vi "input_channel_task.vi"(8 "error in":errorcluster, 10 "Analog Input Channels":T2[](array[typedef])=[{"Input Type"=enum."DAQ", "Channel Name"="Vapor Mass Flow", "Physical Channel"="cDAQ1Mod2/ai5", "Sensor Type"=enum."Mass Flow Rate", "Signal Type"=enum."Current", "Terminal Configuration"=-1, "Minimum Value"=0.004, "Maximum Value"=0.02, "TC Type"=10086, "Sensor Min"=0.0, "Sensor Max"=377.9933, "Sensor Offset"=0.0, "Sensor Unit"=enum."g/s", "Output Unit"=enum."g/s", "Unit Conversion"=1.0, "Active"=TRUE}, {"Input Type"=enum."DAQ", "Channel Name"="Vapor Line Density", "Physical Channel"="cDAQ1Mod2/ai6", "Sensor Type"=enum."Density", "Signal Type"=enum."Current", "Terminal Configuration"=-1, "Minimum Value"=0.004, "Maximum Value"=0.02, "TC Type"=10086, "Sensor Min"=0.0, "Sensor Max"=2.0, "Sensor Offset"=0.0, "Sensor Unit"=enum."g/cm3", "Output Unit"=enum."g/cm3", "Unit Conversion"=1.0, "Active"=TRUE}, {"Input Type"=enum."DAQ", "Channel Name"="Liquid Mass Flow", "Physical Channel"="cDAQ1Mod2/ai3", "Sensor Type"=enum."Mass Flow Rate", "Signal Type"=enum."Current", "Terminal Configuration"=-1, "Minimum Value"=0.004, "Maximum Value"=0.02, "TC Type"=10086, "Sensor Min"=0.0, "Sensor Max"=377.9933, "Sensor Offset"=0.0, "Sensor Unit"=enum."g/s", "Output Unit"=enum."g/s", "Unit Conversion"=1.0, "Active"=TRUE}, {"Input Type"=enum."DAQ", "Channel Name"="Liquid Line Density", "Physical Channel"="cDAQ1Mod2/ai4", "Sensor Type"=enum."Density", "Signal Type"=enum."Current", "Terminal Configuration"=-1, "Minimum Value"=0.004, "Maximum Value"=0.02, "TC Type"=10086, "Sensor Min"=0.0, "Sensor Max"=2.0, "Sensor Offset"=0.0, "Sensor Unit"=enum."g/cm3", "Output Unit"=enum."g/cm3", "Unit Conversion"=1.0, "Active"=TRUE}, {"Input Type"=enum."DAQ", "Channel Name"="Vapor Inlet Pressure DEPR", "Physical Channel"="cDAQ1Mod5/ai1", "Sensor Type"=enum."Absolute Pressure", "Signal Type"=enum."Voltage", "Terminal Configuration"=10078, "Minimum Value"=0.0, "Maximum Value"=5.0, "TC Type"=10086, "Sensor Min"=0.0, "Sensor Max"=50.0, "Sensor Offset"=0.0, "Sensor Unit"=enum."psi", "Output Unit"=enum."Pa", "Unit Conversion"=6894.75729, "Active"=FALSE}, {"Input Type"=enum."DAQ", "Channel Name"="Mega Tank Pressure", "Physical Channel"="cDAQ1Mod5/ai2", "Sensor Type"=enum."Absolute Pressure", "Signal Type"=enum."Voltage", "Terminal Configuration"=10078, "Minimum Value"=0.5, "Maximum Value"=5.5, "TC Type"=10086, "Sensor Min"=0.0, "Sensor Max"=50.0, "Sensor Offset"=0.0, "Sensor Unit"=enum."psi", "Output Unit"=enum."Pa", "Unit Conversion"=6894.75729, "Active"=TRUE}, {"Input Type"=enum."DAQ", "Channel Name"="Separator Pressure", "Physical Channel"="cDAQ1Mod5/ai0", "Sensor Type"=enum."Absolute Pressure", "Signal Type"=enum."Voltage", "Terminal Configuration"=10078, "Minimum Value"=0.0, "Maximum Value"=5.0, "TC Type"=10086, "Sensor Min"=0.0, "Sensor Max"=50.0, "Sensor Offset"=0.0, "Sensor Unit"=enum."psi", "Output Unit"=enum."Pa", "Unit Conversion"=6894.75729, "Active"=TRUE}, {"Input Type"=enum."DAQ", "Channel Name"="Liquid Inlet Pressure", "Physical Channel"="cDAQ1Mod5/ai4", "Sensor Type"=enum."Absolute Pressure", "Signal Type"=enum."Voltage", "Terminal Configuration"=10078, "Minimum Value"=0.0, "Maximum Value"=5.0, "TC Type"=10086, "Sensor Min"=0.0, "Sensor Max"=50.0, "Sensor Offset"=0.0, "Sensor Unit"=enum."psi", "Output Unit"=enum."Pa", "Unit Conversion"=6894.75729, "Active"=TRUE}, {"Input Type"=enum."DAQ", "Channel Name"="Vapor Inlet Pressure ", "Physical Channel"="cDAQ1Mod5/ai3", "Sensor Type"=enum."Absolute Pressure", "Signal Type"=enum."Voltage", "Terminal Configuration"=10078, "Minimum Value"=0.0, "Maximum Value"=5.0, "TC Type"=10086, "Sensor Min"=0.0, "Sensor Max"=50.0, "Sensor Offset"=0.0, "Sensor Unit"=enum."psi", "Output Unit"=enum."Pa", "Unit Conversion"=6894.75729, "Active"=TRUE}, {"Input Type"=enum."DAQ", "Channel Name"="Vapor Inlet Temperature", "Physical Channel"="cDAQ1Mod6/ai1", "Sensor Type"=enum."Temperature", "Signal Type"=enum."Temperature", "Terminal Configuration"=-1, "Minimum Value"=0.0, "Maximum Value"=100.0, "TC Type"=10086, "Sensor Min"=0.0, "Sensor Max"=100.0, "Sensor Offset"=0.0, "Sensor Unit"=enum."C", "Output Unit"=enum."C", "Unit Conversion"=1.0, "Active"=TRUE}, {"Input Type"=enum."DAQ", "Channel Name"="Vapor Inlet Temperature DEPR", "Physical Channel"="cDAQ1Mod7/ai0", "Sensor Type"=enum."Temperature", "Signal Type"=enum."Temperature", "Terminal Configuration"=-1, "Minimum Value"=0.0, "Maximum Value"=100.0, "TC Type"=10086, "Sensor Min"=0.0, "Sensor Max"=100.0, "Sensor Offset"=0.0, "Sensor Unit"=enum."C", "Output Unit"=enum."C", "Unit Conversion"=1.0, "Active"=FALSE}, {"Input Type"=enum."DAQ", "Channel Name"="Mega Tank Temperature", "Physical Channel"="cDAQ1Mod6/ai2", "Sensor Type"=enum."Temperature", "Signal Type"=enum."Temperature", "Terminal Configuration"=-1, "Minimum Value"=0.0, "Maximum Value"=100.0, "TC Type"=10086, "Sensor Min"=0.0, "Sensor Max"=100.0, "Sensor Offset"=0.0, "Sensor Unit"=enum."C", "Output Unit"=enum."C", "Unit Conversion"=1.0, "Active"=TRUE}, {"Input Type"=enum."DAQ", "Channel Name"="Liquid Inlet Temperature", "Physical Channel"="cDAQ1Mod7/ai3", "Sensor Type"=enum."Temperature", "Signal Type"=enum."Temperature", "Terminal Configuration"=-1, "Minimum Value"=0.0, "Maximum Value"=100.0, "TC Type"=10086, "Sensor Min"=0.0, "Sensor Max"=100.0, "Sensor Offset"=0.0, "Sensor Unit"=enum."C", "Output Unit"=enum."C", "Unit Conversion"=1.0, "Active"=TRUE}, {"Input Type"=enum."DAQ", "Channel Name"="Separator Temperature", "Physical Channel"="cDAQ1Mod6/ai0", "Sensor Type"=enum."Temperature", "Signal Type"=enum."Temperature", "Terminal Configuration"=-1, "Minimum Value"=0.0, "Maximum Value"=100.0, "TC Type"=10086, "Sensor Min"=0.0, "Sensor Max"=100.0, "Sensor Offset"=0.0, "Sensor Unit"=enum."C", "Output Unit"=enum."C", "Unit Conversion"=1.0, "Active"=TRUE}, {"Input Type"=enum."DAQ", "Channel Name"="Lower Dev Section Pressure", "Physical Channel"="cDAQ1Mod5/ai6", "Sensor Type"=enum."Absolute Pressure", "Signal Type"=enum."Voltage", "Terminal Configuration"=10078, "Minimum Value"=0.0, "Maximum Value"=5.0, "TC Type"=10086, "Sensor Min"=0.0, "Sensor Max"=60.0, "Sensor Offset"=0.0, "Sensor Unit"=enum."psi", "Output Unit"=enum."Pa", "Unit Conversion"=6894.75729, "Active"=TRUE}, {"Input Type"=enum."DAQ", "Channel Name"="Upper Dev Section Temperature", "Physical Channel"="cDAQ1Mod6/ai3", "Sensor Type"=enum."Temperature", "Signal Type"=enum."Temperature", "Terminal Configuration"=-1, "Minimum Value"=0.0, "Maximum Value"=100.0, "TC Type"=10086, "Sensor Min"=0.0, "Sensor Max"=100.0, "Sensor Offset"=0.0, "Sensor Unit"=enum."C", "Output Unit"=enum."C", "Unit Conversion"=1.0, "Active"=TRUE}, {"Input Type"=enum."DAQ", "Channel Name"="Upper Dev Section Pressure", "Physical Channel"="cDAQ1Mod5/ai5", "Sensor Type"=enum."Absolute Pressure", "Signal Type"=enum."Voltage", "Terminal Configuration"=10078, "Minimum Value"=0.0, "Maximum Value"=5.0, "TC Type"=10086, "Sensor Min"=0.0, "Sensor Max"=60.0, "Sensor Offset"=0.0, "Sensor Unit"=enum."psi", "Output Unit"=enum."Pa", "Unit Conversion"=6894.75729, "Active"=TRUE}, {"Input Type"=enum."DAQ", "Channel Name"="Test Section Temperature", "Physical Channel"="cDAQ1Mod6/ai10", "Sensor Type"=enum."Temperature", "Signal Type"=enum."Temperature", "Terminal Configuration"=-1, "Minimum Value"=0.0, "Maximum Value"=100.0, "TC Type"=10086, "Sensor Min"=0.0, "Sensor Max"=100.0, "Sensor Offset"=0.0, "Sensor Unit"=enum."C", "Output Unit"=enum."C", "Unit Conversion"=1.0, "Active"=TRUE}, {"Input Type"=enum."DAQ", "Channel Name"="Test Section Pressure", "Physical Channel"="cDAQ1Mod5/ai7", "Sensor Type"=enum."Absolute Pressure", "Signal Type"=enum."Voltage", "Terminal Configuration"=10078, "Minimum Value"=0.0, "Maximum Value"=5.0, "TC Type"=10086, "Sensor Min"=0.0, "Sensor Max"=50.0, "Sensor Offset"=0.0, "Sensor Unit"=enum."psi", "Output Unit"=enum."Pa", "Unit Conversion"=6894.75729, "Active"=TRUE}, {"Input Type"=enum."DAQ", "Channel Name"="Dwyer dP DEPR", "Physical Channel"="cDAQ1Mod5/ai9", "Sensor Type"=enum."Differential Pressure", "Signal Type"=enum."Voltage", "Terminal Configuration"=10078, "Minimum Value"=0.05, "Maximum Value"=5.05, "TC Type"=10086, "Sensor Min"=0.0, "Sensor Max"=1.0, "Sensor Offset"=0.0, "Sensor Unit"=enum."psi", "Output Unit"=enum."Pa", "Unit Conversion"=6894.75729, "Active"=FALSE}, {"Input Type"=enum."DAQ", "Channel Name"="Venturi dP", "Physical Channel"="cDAQ1Mod9/ai0", "Sensor Type"=enum."Differential Pressure", "Signal Type"=enum."Current", "Terminal Configuration"=10083, "Minimum Value"=0.00403, "Maximum Value"=0.02, "TC Type"=10086, "Sensor Min"=0.0, "Sensor Max"=10.0, "Sensor Offset"=0.0, "Sensor Unit"=enum."inH2O", "Output Unit"=enum."Pa", "Unit Conversion"=248.84, "Active"=TRUE}, {"Input Type"=enum."DAQ", "Channel Name"="PGminiPressure", "Physical Channel"="cDAQ1Mod5/ai10", "Sensor Type"=enum."Absolute Pressure", "Signal Type"=enum."Voltage", "Terminal Configuration"=10078, "Minimum Value"=0.0, "Maximum Value"=5.0, "TC Type"=10086, "Sensor Min"=0.0, "Sensor Max"=50.0, "Sensor Offset"=0.0, "Sensor Unit"=enum."psi", "Output Unit"=enum."Pa", "Unit Conversion"=6894.75729, "Active"=TRUE}, {"Input Type"=enum."DAQ", "Channel Name"="PGminiTemperature", "Physical Channel"="cDAQ1Mod7/ai6", "Sensor Type"=enum."Temperature", "Signal Type"=enum."Temperature", "Terminal Configuration"=-1, "Minimum Value"=0.0, "Maximum Value"=100.0, "TC Type"=10073, "Sensor Min"=0.0, "Sensor Max"=100.0, "Sensor Offset"=0.0, "Sensor Unit"=enum."C", "Output Unit"=enum."C", "Unit Conversion"=1.0, "Active"=TRUE}, {"Input Type"=enum."DAQ", "Channel Name"="Atmospheric Pressure", "Physical Channel"="cDAQ1Mod5/ai8", "Sensor Type"=enum."Absolute Pressure", "Signal Type"=enum."Voltage", "Terminal Configuration"=10078, "Minimum Value"=1.0, "Maximum Value"=5.0, "TC Type"=10086, "Sensor Min"=0.0, "Sensor Max"=25.0, "Sensor Offset"=0.0, "Sensor Unit"=enum."psi", "Output Unit"=enum."Pa", "Unit Conversion"=6894.75729, "Active"=TRUE}, {"Input Type"=enum."DAQ", "Channel Name"="PG Absolute Pressure", "Physical Channel"="cDAQ1Mod5/ai11", "Sensor Type"=enum."Absolute Pressure", "Signal Type"=enum."Voltage", "Terminal Configuration"=10078, "Minimum Value"=0.0, "Maximum Value"=5.0, "TC Type"=10086, "Sensor Min"=0.0, "Sensor Max"=60.0, "Sensor Offset"=0.0, "Sensor Unit"=enum."psi", "Output Unit"=enum."Pa", "Unit Conversion"=6894.75729, "Active"=TRUE}, {"Input Type"=enum."DAQ", "Channel Name"="Dwyer dP", "Physical Channel"="cDAQ1Mod2/ai7", "Sensor Type"=enum."Differential Pressure", "Signal Type"=enum."Current", "Terminal Configuration"=-1, "Minimum Value"=0.004, "Maximum Value"=0.02, "TC Type"=10086, "Sensor Min"=0.0, "Sensor Max"=500.0, "Sensor Offset"=0.0, "Sensor Unit"=enum."Pa", "Output Unit"=enum."Pa", "Unit Conversion"=1.0, "Active"=TRUE}, {"Input Type"=enum."DAQ", "Channel Name"="Mixing Tee dP DEPR", "Physical Channel"="", "Sensor Type"=enum."Differential Pressure", "Signal Type"=enum."Current", "Terminal Configuration"=-1, "Minimum Value"=0.004, "Maximum Value"=0.02, "TC Type"=10086, "Sensor Min"=0.0, "Sensor Max"=50.0, "Sensor Offset"=0.0, "Sensor Unit"=enum."psi", "Output Unit"=enum."Pa", "Unit Conversion"=6894.75729, "Active"=FALSE}, {"Input Type"=enum."DAQ", "Channel Name"="PG Vapor Temperature", "Physical Channel"="cDAQ1Mod7/ai4", "Sensor Type"=enum."Temperature", "Signal Type"=enum."Temperature", "Terminal Configuration"=-1, "Minimum Value"=0.0, "Maximum Value"=100.0, "TC Type"=10073, "Sensor Min"=0.0, "Sensor Max"=100.0, "Sensor Offset"=0.0, "Sensor Unit"=enum."C", "Output Unit"=enum."C", "Unit Conversion"=1.0, "Active"=TRUE}, {"Input Type"=enum."DAQ", "Channel Name"="PG Liquid Temperature", "Physical Channel"="cDAQ1Mod7/ai5", "Sensor Type"=enum."Temperature", "Signal Type"=enum."Temperature", "Terminal Configuration"=-1, "Minimum Value"=0.0, "Maximum Value"=100.0, "TC Type"=10073, "Sensor Min"=0.0, "Sensor Max"=100.0, "Sensor Offset"=0.0, "Sensor Unit"=enum."C", "Output Unit"=enum."C", "Unit Conversion"=1.0, "Active"=TRUE}, {"Input Type"=enum."DAQ", "Channel Name"="Window 1 to 4 dP", "Physical Channel"="cDAQ1Mod2/ai2", "Sensor Type"=enum."Differential Pressure", "Signal Type"=enum."Current", "Terminal Configuration"=-1, "Minimum Value"=0.004, "Maximum Value"=0.02, "TC Type"=10086, "Sensor Min"=0.0, "Sensor Max"=20.0, "Sensor Offset"=0.0, "Sensor Unit"=enum."inH2O", "Output Unit"=enum."Pa", "Unit Conversion"=248.84, "Active"=TRUE}, {"Input Type"=enum."DAQ", "Channel Name"="Window 1 to 7 dP", "Physical Channel"="cDAQ1Mod2/ai1", "Sensor Type"=enum."Differential Pressure", "Signal Type"=enum."Current", "Terminal Configuration"=-1, "Minimum Value"=0.004, "Maximum Value"=0.02, "TC Type"=10086, "Sensor Min"=0.0, "Sensor Max"=20.0, "Sensor Offset"=0.0, "Sensor Unit"=enum."inH2O", "Output Unit"=enum."Pa", "Unit Conversion"=248.84, "Active"=TRUE}, {"Input Type"=enum."DAQ", "Channel Name"="Window 1 to 7 Fast dP", "Physical Channel"="cDAQ1Mod2/ai0", "Sensor Type"=enum."Differential Pressure", "Signal Type"=enum."Current", "Terminal Configuration"=-1, "Minimum Value"=0.004, "Maximum Value"=0.02, "TC Type"=10086, "Sensor Min"=0.0, "Sensor Max"=2.5, "Sensor Offset"=0.0, "Sensor Unit"=enum."psi", "Output Unit"=enum."Pa", "Unit Conversion"=6894.75729, "Active"=TRUE}, {"Input Type"=enum."DAQ", "Channel Name"="Camera Voltage", "Physical Channel"="cDAQ1Mod8/ai0", "Sensor Type"=enum."Other", "Signal Type"=enum."Voltage", "Terminal Configuration"=10106, "Minimum Value"=0.0, "Maximum Value"=10.0, "TC Type"=10086, "Sensor Min"=0.0, "Sensor Max"=50.0, "Sensor Offset"=0.0, "Sensor Unit"=enum."Volt", "Output Unit"=enum."Volt", "Unit Conversion"=1.0, "Active"=TRUE}, {"Input Type"=enum."DAQ", "Channel Name"="Tinlet", "Physical Channel"="cDAQ1Mod6/ai4", "Sensor Type"=enum."Temperature", "Signal Type"=enum."Temperature", "Terminal Configuration"=-1, "Minimum Value"=0.0, "Maximum Value"=100.0, "TC Type"=10055, "Sensor Min"=-0.432, "Sensor Max"=99.438, "Sensor Offset"=0.0, "Sensor Unit"=enum."C", "Output Unit"=enum."C", "Unit Conversion"=1.0, "Active"=TRUE}, {"Input Type"=enum."DAQ", "Channel Name"="Tsectwo", "Physical Channel"="cDAQ1Mod6/ai5", "Sensor Type"=enum."Temperature", "Signal Type"=enum."Temperature", "Terminal Configuration"=-1, "Minimum Value"=0.0, "Maximum Value"=100.0, "TC Type"=10055, "Sensor Min"=-0.3803, "Sensor Max"=99.4597, "Sensor Offset"=0.0, "Sensor Unit"=enum."C", "Output Unit"=enum."C", "Unit Conversion"=1.0, "Active"=TRUE}, {"Input Type"=enum."DAQ", "Channel Name"="TS Window 1 Absolute Pressure", "Physical Channel"="cDAQ1Mod5/ai12", "Sensor Type"=enum."Absolute Pressure", "Signal Type"=enum."Voltage", "Terminal Configuration"=10078, "Minimum Value"=0.0, "Maximum Value"=5.0, "TC Type"=10086, "Sensor Min"=0.0, "Sensor Max"=50.0, "Sensor Offset"=0.0, "Sensor Unit"=enum."psi", "Output Unit"=enum."Pa", "Unit Conversion"=6894.75729, "Active"=TRUE}, {"Input Type"=enum."DAQ", "Channel Name"="TS Window 7 Absolute Pressure", "Physical Channel"="cDAQ1Mod5/ai13", "Sensor Type"=enum."Absolute Pressure", "Signal Type"=enum."Voltage", "Terminal Configuration"=10078, "Minimum Value"=0.0, "Maximum Value"=5.0, "TC Type"=10086, "Sensor Min"=0.0, "Sensor Max"=50.0, "Sensor Offset"=0.0, "Sensor Unit"=enum."psi", "Output Unit"=enum."Pa", "Unit Conversion"=6894.75729, "Active"=TRUE}, {"Input Type"=enum."DAQ", "Channel Name"="Liquid Main Diode", "Physical Channel"="cDAQ1Mod10/ai0", "Sensor Type"=enum."Other", "Signal Type"=enum."Voltage", "Terminal Configuration"=10106, "Minimum Value"=0.0, "Maximum Value"=10.0, "TC Type"=10086, "Sensor Min"=0.0, "Sensor Max"=10.0, "Sensor Offset"=0.0, "Sensor Unit"=enum."Volt", "Output Unit"=enum."Volt", "Unit Conversion"=1.0, "Active"=TRUE}, {"Input Type"=enum."DAQ", "Channel Name"="Liquid Control Diode", "Physical Channel"="cDAQ1Mod10/ai1", "Sensor Type"=enum."Other", "Signal Type"=enum."Voltage", "Terminal Configuration"=10106, "Minimum Value"=0.0, "Maximum Value"=10.0, "TC Type"=10086, "Sensor Min"=0.0, "Sensor Max"=10.0, "Sensor Offset"=0.0, "Sensor Unit"=enum."Volt", "Output Unit"=enum."Volt", "Unit Conversion"=1.0, "Active"=TRUE}, {"Input Type"=enum."DAQ", "Channel Name"="Vapor Main Diode", "Physical Channel"="cDAQ1Mod10/ai2", "Sensor Type"=enum."Other", "Signal Type"=enum."Voltage", "Terminal Configuration"=10106, "Minimum Value"=0.0, "Maximum Value"=10.0, "TC Type"=10086, "Sensor Min"=0.0, "Sensor Max"=10.0, "Sensor Offset"=0.0, "Sensor Unit"=enum."Volt", "Output Unit"=enum."Volt", "Unit Conversion"=1.0, "Active"=TRUE}, {"Input Type"=enum."DAQ", "Channel Name"="Vapor Control Diode", "Physical Channel"="cDAQ1Mod10/ai3", "Sensor Type"=enum."Other", "Signal Type"=enum."Voltage", "Terminal Configuration"=10106, "Minimum Value"=0.0, "Maximum Value"=10.0, "TC Type"=10086, "Sensor Min"=0.0, "Sensor Max"=10.0, "Sensor Offset"=0.0, "Sensor Unit"=enum."Volt", "Output Unit"=enum."Volt", "Unit Conversion"=1.0, "Active"=TRUE}, {"Input Type"=enum."DAQ", "Channel Name"="TS Exterior Temperature", "Physical Channel"="cDAQ1Mod6/ai6", "Sensor Type"=enum."Temperature", "Signal Type"=enum."Temperature", "Terminal Configuration"=-1, "Minimum Value"=0.0, "Maximum Value"=100.0, "TC Type"=10073, "Sensor Min"=-0.2775, "Sensor Max"=100.1225, "Sensor Offset"=0.0, "Sensor Unit"=enum."C", "Output Unit"=enum."C", "Unit Conversion"=1.0, "Active"=TRUE}, {"Input Type"=enum."DAQ", "Channel Name"="PG Supply Temperature", "Physical Channel"="cDAQ1Mod6/ai7", "Sensor Type"=enum."Temperature", "Signal Type"=enum."Temperature", "Terminal Configuration"=-1, "Minimum Value"=0.0, "Maximum Value"=100.0, "TC Type"=10073, "Sensor Min"=0.0, "Sensor Max"=100.0, "Sensor Offset"=0.0, "Sensor Unit"=enum."C", "Output Unit"=enum."C", "Unit Conversion"=1.0, "Active"=TRUE}, {"Input Type"=enum."DAQ", "Channel Name"="Post Mixing Tee Temperature", "Physical Channel"="cDAQ1Mod7/ai2", "Sensor Type"=enum."Temperature", "Signal Type"=enum."Temperature", "Terminal Configuration"=-1, "Minimum Value"=0.0, "Maximum Value"=100.0, "TC Type"=10073, "Sensor Min"=0.0, "Sensor Max"=1000.0, "Sensor Offset"=0.0, "Sensor Unit"=enum."Volt", "Output Unit"=enum."Volt", "Unit Conversion"=1.0, "Active"=TRUE}, {"Input Type"=enum."DAQ", "Channel Name"="Tsecthree", "Physical Channel"="cDAQ1Mod6/ai8", "Sensor Type"=enum."Temperature", "Signal Type"=enum."Temperature", "Terminal Configuration"=-1, "Minimum Value"=0.0, "Maximum Value"=100.0, "TC Type"=10055, "Sensor Min"=-0.2553, "Sensor Max"=99.6347, "Sensor Offset"=0.0, "Sensor Unit"=enum."C", "Output Unit"=enum."C", "Unit Conversion"=1.0, "Active"=TRUE}, {"Input Type"=enum."DAQ", "Channel Name"="Toutlet", "Physical Channel"="cDAQ1Mod6/ai9", "Sensor Type"=enum."Temperature", "Signal Type"=enum."Temperature", "Terminal Configuration"=-1, "Minimum Value"=0.0, "Maximum Value"=100.0, "TC Type"=10055, "Sensor Min"=-0.1957, "Sensor Max"=99.8043, "Sensor Offset"=0.0, "Sensor Unit"=enum."C", "Output Unit"=enum."C", "Unit Conversion"=1.0, "Active"=TRUE}, {"Input Type"=enum."DAQ", "Channel Name"="TS Exterior T 1", "Physical Channel"="cDAQ1Mod9/ai0", "Sensor Type"=enum."Temperature", "Signal Type"=enum."Temperature", "Terminal Configuration"=-1, "Minimum Value"=0.0, "Maximum Value"=100.0, "TC Type"=10055, "Sensor Min"=0.39257, "Sensor Max"=101.06323, "Sensor Offset"=0.0, "Sensor Unit"=enum."C", "Output Unit"=enum."C", "Unit Conversion"=1.0, "Active"=TRUE}, {"Input Type"=enum."DAQ", "Channel Name"="TS Exterior T 2", "Physical Channel"="cDAQ1Mod9/ai1", "Sensor Type"=enum."Temperature", "Signal Type"=enum."Temperature", "Terminal Configuration"=-1, "Minimum Value"=0.0, "Maximum Value"=100.0, "TC Type"=10055, "Sensor Min"=0.47457, "Sensor Max"=101.13515, "Sensor Offset"=0.0, "Sensor Unit"=enum."C", "Output Unit"=enum."C", "Unit Conversion"=1.0, "Active"=TRUE}, {"Input Type"=enum."DAQ", "Channel Name"="TS Exterior T 3", "Physical Channel"="cDAQ1Mod9/ai2", "Sensor Type"=enum."Temperature", "Signal Type"=enum."Temperature", "Terminal Configuration"=-1, "Minimum Value"=0.0, "Maximum Value"=100.0, "TC Type"=10055, "Sensor Min"=0.65169, "Sensor Max"=101.29195, "Sensor Offset"=0.0, "Sensor Unit"=enum."C", "Output Unit"=enum."C", "Unit Conversion"=1.0, "Active"=TRUE}, {"Input Type"=enum."DAQ", "Channel Name"="TS Exterior T 4", "Physical Channel"="cDAQ1Mod9/ai3", "Sensor Type"=enum."Temperature", "Signal Type"=enum."Temperature", "Terminal Configuration"=-1, "Minimum Value"=0.0, "Maximum Value"=100.0, "TC Type"=10055, "Sensor Min"=0.85075, "Sensor Max"=101.45817, "Sensor Offset"=0.0, "Sensor Unit"=enum."C", "Output Unit"=enum."C", "Unit Conversion"=1.0, "Active"=TRUE}, {"Input Type"=enum."DAQ", "Channel Name"="TS Exterior T 5", "Physical Channel"="cDAQ1Mod9/ai0", "Sensor Type"=enum."Temperature", "Signal Type"=enum."Temperature", "Terminal Configuration"=-1, "Minimum Value"=0.0, "Maximum Value"=100.0, "TC Type"=10055, "Sensor Min"=0.30495, "Sensor Max"=100.97891, "Sensor Offset"=0.0, "Sensor Unit"=enum."C", "Output Unit"=enum."C", "Unit Conversion"=1.0, "Active"=TRUE}] {"Unit Conversion" format="%0.5f"; "TC Type" items=["J"=10072, "K"=10073, "N"=10077, "R"=10082, "S"=10085, "T"=10086, "B"=10047, "E"=10055]; "Sensor Offset" format="%0.5f"; "Sensor Max" format="%0.5f"; "Sensor Min" format="%0.5f"; "Maximum Value" format="%.6f"; "Minimum Value" format="%.6f"; "Terminal Configuration" items=["Default"=-1, "RSE"=10083, "NRSE"=10078, "Differential"=10106, "Pseudodifferential"=12529]}) -> (0 "error out":errorcluster, 2 "Active Analog Channel-Data Packages":T1[](array[typedef])=[{"Analog Input Channel"={"Input Type"=enum."DAQ", "Channel Name"="Vapor Mass Flow", "Physical Channel"="cDAQ1Mod2/ai5", "Sensor Type"=enum."Mass Flow Rate", "Signal Type"=enum."Current", "Terminal Configuration"=-1, "Minimum Value"=0.004, "Maximum Value"=0.02, "TC Type"=10086, "Sensor Min"=0.0, "Sensor Max"=377.9933, "Sensor Offset"=0.0, "Sensor Unit"=enum."g/s", "Output Unit"=enum."g/s", "Unit Conversion"=1.0, "Active"=TRUE}, "Analog Data"={"Label"="VaporMassFlow", "Offset"=0.0, "Raw"=[], "Converted"=[], "Average"=0.0, "Formula To Output"="(23624.581250*(x-0.004000)+0.000000)*1.000000", "Formula From Output"="(y/1.000000-0.000000)/23624.581250+0.004000"}}, {"Analog Input Channel"={"Input Type"=enum."DAQ", "Channel Name"="Vapor Line Density", "Physical Channel"="cDAQ1Mod2/ai6", "Sensor Type"=enum."Density", "Signal Type"=enum."Current", "Terminal Configuration"=-1, "Minimum Value"=0.004, "Maximum Value"=0.02, "TC Type"=10086, "Sensor Min"=0.0, "Sensor Max"=2.0, "Sensor Offset"=0.0, "Sensor Unit"=enum."g/cm3", "Output Unit"=enum."g/cm3", "Unit Conversion"=1.0, "Active"=TRUE}, "Analog Data"={"Label"="VaporLineDensity", "Offset"=0.0, "Raw"=[], "Converted"=[], "Average"=0.0, "Formula To Output"="(125.000000*(x-0.004000)+0.000000)*1.000000", "Formula From Output"="(y/1.000000-0.000000)/125.000000+0.004000"}}, {"Analog Input Channel"={"Input Type"=enum."DAQ", "Channel Name"="Liquid Mass Flow", "Physical Channel"="cDAQ1Mod2/ai3", "Sensor Type"=enum."Mass Flow Rate", "Signal Type"=enum."Current", "Terminal Configuration"=-1, "Minimum Value"=0.004, "Maximum Value"=0.02, "TC Type"=10086, "Sensor Min"=0.0, "Sensor Max"=377.9933, "Sensor Offset"=0.0, "Sensor Unit"=enum."g/s", "Output Unit"=enum."g/s", "Unit Conversion"=1.0, "Active"=TRUE}, "Analog Data"={"Label"="LiquidMassFlow", "Offset"=0.0, "Raw"=[], "Converted"=[], "Average"=0.0, "Formula To Output"="(23624.581250*(x-0.004000)+0.000000)*1.000000", "Formula From Output"="(y/1.000000-0.000000)/23624.581250+0.004000"}}, {"Analog Input Channel"={"Input Type"=enum."DAQ", "Channel Name"="Liquid Line Density", "Physical Channel"="cDAQ1Mod2/ai4", "Sensor Type"=enum."Density", "Signal Type"=enum."Current", "Terminal Configuration"=-1, "Minimum Value"=0.004, "Maximum Value"=0.02, "TC Type"=10086, "Sensor Min"=0.0, "Sensor Max"=2.0, "Sensor Offset"=0.0, "Sensor Unit"=enum."g/cm3", "Output Unit"=enum."g/cm3", "Unit Conversion"=1.0, "Active"=TRUE}, "Analog Data"={"Label"="LiquidLineDensity", "Offset"=0.0, "Raw"=[], "Converted"=[], "Average"=0.0, "Formula To Output"="(125.000000*(x-0.004000)+0.000000)*1.000000", "Formula From Output"="(y/1.000000-0.000000)/125.000000+0.004000"}}, {"Analog Input Channel"={"Input Type"=enum."DAQ", "Channel Name"="Vapor Inlet Pressure", "Physical Channel"="cDAQ1Mod5/ai1", "Sensor Type"=enum."Absolute Pressure", "Signal Type"=enum."Voltage", "Terminal Configuration"=10078, "Minimum Value"=0.0, "Maximum Value"=5.0, "TC Type"=10086, "Sensor Min"=0.0, "Sensor Max"=50.0, "Sensor Offset"=0.0, "Sensor Unit"=enum."psi", "Output Unit"=enum."Pa", "Unit Conversion"=6894.75729, "Active"=TRUE}, "Analog Data"={"Label"="VaporInletPressure", "Offset"=0.0, "Raw"=[], "Converted"=[], "Average"=0.0, "Formula To Output"="(10.000000*(x-0.000000)+0.000000)*6894.757290", "Formula From Output"="(y/6894.757290-0.000000)/10.000000+0.000000"}}, {"Analog Input Channel"={"Input Type"=enum."DAQ", "Channel Name"="Mega Tank Pressure", "Physical Channel"="cDAQ1Mod5/ai2", "Sensor Type"=enum."Absolute Pressure", "Signal Type"=enum."Voltage", "Terminal Configuration"=10078, "Minimum Value"=0.0, "Maximum Value"=5.0, "TC Type"=10086, "Sensor Min"=0.0, "Sensor Max"=50.0, "Sensor Offset"=0.0, "Sensor Unit"=enum."psi", "Output Unit"=enum."Pa", "Unit Conversion"=6894.75729, "Active"=TRUE}, "Analog Data"={"Label"="MegaTankPressure", "Offset"=0.0, "Raw"=[], "Converted"=[], "Average"=0.0, "Formula To Output"="(10.000000*(x-0.000000)+0.000000)*6894.757290", "Formula From Output"="(y/6894.757290-0.000000)/10.000000+0.000000"}}, {"Analog Input Channel"={"Input Type"=enum."DAQ", "Channel Name"="Separator Pressure", "Physical Channel"="cDAQ1Mod5/ai0", "Sensor Type"=enum."Absolute Pressure", "Signal Type"=enum."Voltage", "Terminal Configuration"=10078, "Minimum Value"=0.0, "Maximum Value"=5.0, "TC Type"=10086, "Sensor Min"=0.0, "Sensor Max"=50.0, "Sensor Offset"=0.0, "Sensor Unit"=enum."psi", "Output Unit"=enum."Pa", "Unit Conversion"=6894.75729, "Active"=TRUE}, "Analog Data"={"Label"="SeparatorPressure", "Offset"=0.0, "Raw"=[], "Converted"=[], "Average"=0.0, "Formula To Output"="(10.000000*(x-0.000000)+0.000000)*6894.757290", "Formula From Output"="(y/6894.757290-0.000000)/10.000000+0.000000"}}, {"Analog Input Channel"={"Input Type"=enum."DAQ", "Channel Name"="Liquid Inlet Pressure", "Physical Channel"="cDAQ1Mod5/ai4", "Sensor Type"=enum."Absolute Pressure", "Signal Type"=enum."Voltage", "Terminal Configuration"=10078, "Minimum Value"=0.0, "Maximum Value"=5.0, "TC Type"=10086, "Sensor Min"=0.0, "Sensor Max"=50.0, "Sensor Offset"=0.0, "Sensor Unit"=enum."psi", "Output Unit"=enum."Pa", "Unit Conversion"=6894.75729, "Active"=TRUE}, "Analog Data"={"Label"="LiquidInletPressure", "Offset"=0.0, "Raw"=[], "Converted"=[], "Average"=0.0, "Formula To Output"="(10.000000*(x-0.000000)+0.000000)*6894.757290", "Formula From Output"="(y/6894.757290-0.000000)/10.000000+0.000000"}}, {"Analog Input Channel"={"Input Type"=enum."DAQ", "Channel Name"="Vapor Inlet Temperature", "Physical Channel"="cDAQ1Mod6/ai1", "Sensor Type"=enum."Temperature", "Signal Type"=enum."Temperature", "Terminal Configuration"=-1, "Minimum Value"=0.0, "Maximum Value"=100.0, "TC Type"=10086, "Sensor Min"=0.0, "Sensor Max"=100.0, "Sensor Offset"=0.0, "Sensor Unit"=enum."C", "Output Unit"=enum."C", "Unit Conversion"=1.0, "Active"=TRUE}, "Analog Data"={"Label"="VaporInletTemperature", "Offset"=0.0, "Raw"=[], "Converted"=[], "Average"=0.0, "Formula To Output"="(1.000000*(x-0.000000)+0.000000)*1.000000", "Formula From Output"="(y/1.000000-0.000000)/1.000000+0.000000"}}, {"Analog Input Channel"={"Input Type"=enum."DAQ", "Channel Name"="Mega Tank Temperature", "Physical Channel"="cDAQ1Mod6/ai2", "Sensor Type"=enum."Temperature", "Signal Type"=enum."Temperature", "Terminal Configuration"=-1, "Minimum Value"=0.0, "Maximum Value"=100.0, "TC Type"=10086, "Sensor Min"=0.0, "Sensor Max"=100.0, "Sensor Offset"=0.0, "Sensor Unit"=enum."C", "Output Unit"=enum."C", "Unit Conversion"=1.0, "Active"=TRUE}, "Analog Data"={"Label"="MegaTankTemperature", "Offset"=0.0, "Raw"=[], "Converted"=[], "Average"=0.0, "Formula To Output"="(1.000000*(x-0.000000)+0.000000)*1.000000", "Formula From Output"="(y/1.000000-0.000000)/1.000000+0.000000"}}, {"Analog Input Channel"={"Input Type"=enum."DAQ", "Channel Name"="Liquid Inlet Temperature", "Physical Channel"="cDAQ1Mod7/ai3", "Sensor Type"=enum."Temperature", "Signal Type"=enum."Temperature", "Terminal Configuration"=-1, "Minimum Value"=0.0, "Maximum Value"=100.0, "TC Type"=10086, "Sensor Min"=0.0, "Sensor Max"=100.0, "Sensor Offset"=0.0, "Sensor Unit"=enum."C", "Output Unit"=enum."C", "Unit Conversion"=1.0, "Active"=TRUE}, "Analog Data"={"Label"="LiquidInletTemperature", "Offset"=0.0, "Raw"=[], "Converted"=[], "Average"=0.0, "Formula To Output"="(1.000000*(x-0.000000)+0.000000)*1.000000", "Formula From Output"="(y/1.000000-0.000000)/1.000000+0.000000"}}, {"Analog Input Channel"={"Input Type"=enum."DAQ", "Channel Name"="Separator Temperature", "Physical Channel"="cDAQ1Mod6/ai0", "Sensor Type"=enum."Temperature", "Signal Type"=enum."Temperature", "Terminal Configuration"=-1, "Minimum Value"=0.0, "Maximum Value"=100.0, "TC Type"=10086, "Sensor Min"=0.0, "Sensor Max"=100.0, "Sensor Offset"=0.0, "Sensor Unit"=enum."C", "Output Unit"=enum."C", "Unit Conversion"=1.0, "Active"=TRUE}, "Analog Data"={"Label"="SeparatorTemperature", "Offset"=0.0, "Raw"=[], "Converted"=[], "Average"=0.0, "Formula To Output"="(1.000000*(x-0.000000)+0.000000)*1.000000", "Formula From Output"="(y/1.000000-0.000000)/1.000000+0.000000"}}, {"Analog Input Channel"={"Input Type"=enum."DAQ", "Channel Name"="Lower Dev Section Pressure", "Physical Channel"="cDAQ1Mod5/ai6", "Sensor Type"=enum."Absolute Pressure", "Signal Type"=enum."Voltage", "Terminal Configuration"=10078, "Minimum Value"=0.0, "Maximum Value"=5.0, "TC Type"=10086, "Sensor Min"=0.0, "Sensor Max"=50.0, "Sensor Offset"=0.0, "Sensor Unit"=enum."psi", "Output Unit"=enum."Pa", "Unit Conversion"=6894.75729, "Active"=TRUE}, "Analog Data"={"Label"="LowerDevSectionPressure", "Offset"=0.0, "Raw"=[], "Converted"=[], "Average"=0.0, "Formula To Output"="(10.000000*(x-0.000000)+0.000000)*6894.757290", "Formula From Output"="(y/6894.757290-0.000000)/10.000000+0.000000"}}, {"Analog Input Channel"={"Input Type"=enum."DAQ", "Channel Name"="Upper Dev Section Temperature", "Physical Channel"="cDAQ1Mod6/ai3", "Sensor Type"=enum."Temperature", "Signal Type"=enum."Temperature", "Terminal Configuration"=-1, "Minimum Value"=0.0, "Maximum Value"=100.0, "TC Type"=10086, "Sensor Min"=0.0, "Sensor Max"=100.0, "Sensor Offset"=0.0, "Sensor Unit"=enum."C", "Output Unit"=enum."C", "Unit Conversion"=1.0, "Active"=TRUE}, "Analog Data"={"Label"="UpperDevSectionTemperature", "Offset"=0.0, "Raw"=[], "Converted"=[], "Average"=0.0, "Formula To Output"="(1.000000*(x-0.000000)+0.000000)*1.000000", "Formula From Output"="(y/1.000000-0.000000)/1.000000+0.000000"}}, {"Analog Input Channel"={"Input Type"=enum."DAQ", "Channel Name"="Upper Dev Section Pressure", "Physical Channel"="cDAQ1Mod5/ai5", "Sensor Type"=enum."Absolute Pressure", "Signal Type"=enum."Voltage", "Terminal Configuration"=10078, "Minimum Value"=0.0, "Maximum Value"=5.0, "TC Type"=10086, "Sensor Min"=0.0, "Sensor Max"=60.0, "Sensor Offset"=0.0, "Sensor Unit"=enum."psi", "Output Unit"=enum."Pa", "Unit Conversion"=6894.75729, "Active"=TRUE}, "Analog Data"={"Label"="UpperDevSectionPressure", "Offset"=0.0, "Raw"=[], "Converted"=[], "Average"=0.0, "Formula To Output"="(12.000000*(x-0.000000)+0.000000)*6894.757290", "Formula From Output"="(y/6894.757290-0.000000)/12.000000+0.000000"}}, {"Analog Input Channel"={"Input Type"=enum."DAQ", "Channel Name"="Test Section Temperature", "Physical Channel"="cDAQ1Mod6/ai10", "Sensor Type"=enum."Temperature", "Signal Type"=enum."Temperature", "Terminal Configuration"=-1, "Minimum Value"=0.0, "Maximum Value"=100.0, "TC Type"=10086, "Sensor Min"=0.0, "Sensor Max"=100.0, "Sensor Offset"=0.0, "Sensor Unit"=enum."C", "Output Unit"=enum."C", "Unit Conversion"=1.0, "Active"=TRUE}, "Analog Data"={"Label"="TestSectionTemperature", "Offset"=0.0, "Raw"=[], "Converted"=[], "Average"=0.0, "Formula To Output"="(1.000000*(x-0.000000)+0.000000)*1.000000", "Formula From Output"="(y/1.000000-0.000000)/1.000000+0.000000"}}, {"Analog Input Channel"={"Input Type"=enum."DAQ", "Channel Name"="Test Section Pressure", "Physical Channel"="cDAQ1Mod5/ai7", "Sensor Type"=enum."Absolute Pressure", "Signal Type"=enum."Voltage", "Terminal Configuration"=10078, "Minimum Value"=0.0, "Maximum Value"=5.0, "TC Type"=10086, "Sensor Min"=0.0, "Sensor Max"=50.0, "Sensor Offset"=0.0, "Sensor Unit"=enum."psi", "Output Unit"=enum."Pa", "Unit Conversion"=6894.75729, "Active"=TRUE}, "Analog Data"={"Label"="TestSectionPressure", "Offset"=0.0, "Raw"=[], "Converted"=[], "Average"=0.0, "Formula To Output"="(10.000000*(x-0.000000)+0.000000)*6894.757290", "Formula From Output"="(y/6894.757290-0.000000)/10.000000+0.000000"}}, {"Analog Input Channel"={"Input Type"=enum."DAQ", "Channel Name"="Dwyer dP", "Physical Channel"="cDAQ1Mod5/ai9", "Sensor Type"=enum."Differential Pressure", "Signal Type"=enum."Voltage", "Terminal Configuration"=10078, "Minimum Value"=0.05, "Maximum Value"=5.05, "TC Type"=10086, "Sensor Min"=0.0, "Sensor Max"=1.0, "Sensor Offset"=0.0, "Sensor Unit"=enum."psi", "Output Unit"=enum."Pa", "Unit Conversion"=6894.75729, "Active"=TRUE}, "Analog Data"={"Label"="DwyerdP", "Offset"=0.0, "Raw"=[], "Converted"=[], "Average"=0.0, "Formula To Output"="(0.200000*(x-0.050000)+0.000000)*6894.757290", "Formula From Output"="(y/6894.757290-0.000000)/0.200000+0.050000"}}, {"Analog Input Channel"={"Input Type"=enum."DAQ", "Channel Name"="Venturi dP", "Physical Channel"="cDAQ1Mod9/ai0", "Sensor Type"=enum."Differential Pressure", "Signal Type"=enum."Current", "Terminal Configuration"=10083, "Minimum Value"=0.00403, "Maximum Value"=0.02, "TC Type"=10086, "Sensor Min"=0.0, "Sensor Max"=10.0, "Sensor Offset"=0.0, "Sensor Unit"=enum."inH2O", "Output Unit"=enum."Pa", "Unit Conversion"=248.84, "Active"=TRUE}, "Analog Data"={"Label"="VenturidP", "Offset"=0.0, "Raw"=[], "Converted"=[], "Average"=0.0, "Formula To Output"="(626.174076*(x-0.004030)+0.000000)*248.840000", "Formula From Output"="(y/248.840000-0.000000)/626.174076+0.004030"}}, {"Analog Input Channel"={"Input Type"=enum."DAQ", "Channel Name"="PG inlet-Mixing Tee Pressure", "Physical Channel"="cDAQ1Mod5/ai10", "Sensor Type"=enum."Absolute Pressure", "Signal Type"=enum."Voltage", "Terminal Configuration"=10078, "Minimum Value"=0.0, "Maximum Value"=5.0, "TC Type"=10086, "Sensor Min"=0.0, "Sensor Max"=50.0, "Sensor Offset"=0.0, "Sensor Unit"=enum."psi", "Output Unit"=enum."Pa", "Unit Conversion"=6894.75729, "Active"=TRUE}, "Analog Data"={"Label"="PGinlet-MixingTeePressure", "Offset"=0.0, "Raw"=[], "Converted"=[], "Average"=0.0, "Formula To Output"="(10.000000*(x-0.000000)+0.000000)*6894.757290", "Formula From Output"="(y/6894.757290-0.000000)/10.000000+0.000000"}}, {"Analog Input Channel"={"Input Type"=enum."DAQ", "Channel Name"="PG inlet-Mixing Tee Temperature", "Physical Channel"="cDAQ1Mod7/ai6", "Sensor Type"=enum."Temperature", "Signal Type"=enum."Temperature", "Terminal Configuration"=-1, "Minimum Value"=0.0, "Maximum Value"=100.0, "TC Type"=10073, "Sensor Min"=0.0, "Sensor Max"=100.0, "Sensor Offset"=0.0, "Sensor Unit"=enum."C", "Output Unit"=enum."C", "Unit Conversion"=1.0, "Active"=TRUE}, "Analog Data"={"Label"="PGinlet-MixingTeeTemperature", "Offset"=0.0, "Raw"=[], "Converted"=[], "Average"=0.0, "Formula To Output"="(1.000000*(x-0.000000)+0.000000)*1.000000", "Formula From Output"="(y/1.000000-0.000000)/1.000000+0.000000"}}, {"Analog Input Channel"={"Input Type"=enum."DAQ", "Channel Name"="Atmospheric Pressure", "Physical Channel"="cDAQ1Mod5/ai8", "Sensor Type"=enum."Absolute Pressure", "Signal Type"=enum."Voltage", "Terminal Configuration"=10078, "Minimum Value"=1.0, "Maximum Value"=5.0, "TC Type"=10086, "Sensor Min"=0.0, "Sensor Max"=25.0, "Sensor Offset"=0.0, "Sensor Unit"=enum."psi", "Output Unit"=enum."Pa", "Unit Conversion"=6894.75729, "Active"=TRUE}, "Analog Data"={"Label"="AtmosphericPressure", "Offset"=0.0, "Raw"=[], "Converted"=[], "Average"=0.0, "Formula To Output"="(6.250000*(x-1.000000)+0.000000)*6894.757290", "Formula From Output"="(y/6894.757290-0.000000)/6.250000+1.000000"}}, {"Analog Input Channel"={"Input Type"=enum."DAQ", "Channel Name"="PG Absolute Pressure", "Physical Channel"="cDAQ1Mod5/ai11", "Sensor Type"=enum."Absolute Pressure", "Signal Type"=enum."Voltage", "Terminal Configuration"=10078, "Minimum Value"=0.0, "Maximum Value"=5.0, "TC Type"=10086, "Sensor Min"=0.0, "Sensor Max"=60.0, "Sensor Offset"=0.0, "Sensor Unit"=enum."psi", "Output Unit"=enum."Pa", "Unit Conversion"=6894.75729, "Active"=TRUE}, "Analog Data"={"Label"="PGAbsolutePressure", "Offset"=0.0, "Raw"=[], "Converted"=[], "Average"=0.0, "Formula To Output"="(12.000000*(x-0.000000)+0.000000)*6894.757290", "Formula From Output"="(y/6894.757290-0.000000)/12.000000+0.000000"}}, {"Analog Input Channel"={"Input Type"=enum."DAQ", "Channel Name"="PG Vapor Temperature", "Physical Channel"="cDAQ1Mod7/ai4", "Sensor Type"=enum."Temperature", "Signal Type"=enum."Temperature", "Terminal Configuration"=-1, "Minimum Value"=0.0, "Maximum Value"=100.0, "TC Type"=10073, "Sensor Min"=0.0, "Sensor Max"=100.0, "Sensor Offset"=0.0, "Sensor Unit"=enum."C", "Output Unit"=enum."C", "Unit Conversion"=1.0, "Active"=TRUE}, "Analog Data"={"Label"="PGVaporTemperature", "Offset"=0.0, "Raw"=[], "Converted"=[], "Average"=0.0, "Formula To Output"="(1.000000*(x-0.000000)+0.000000)*1.000000", "Formula From Output"="(y/1.000000-0.000000)/1.000000+0.000000"}}, {"Analog Input Channel"={"Input Type"=enum."DAQ", "Channel Name"="PG Liquid Temperature", "Physical Channel"="cDAQ1Mod7/ai5", "Sensor Type"=enum."Temperature", "Signal Type"=enum."Temperature", "Terminal Configuration"=-1, "Minimum Value"=0.0, "Maximum Value"=100.0, "TC Type"=10073, "Sensor Min"=0.0, "Sensor Max"=100.0, "Sensor Offset"=0.0, "Sensor Unit"=enum."C", "Output Unit"=enum."C", "Unit Conversion"=1.0, "Active"=TRUE}, "Analog Data"={"Label"="PGLiquidTemperature", "Offset"=0.0, "Raw"=[], "Converted"=[], "Average"=0.0, "Formula To Output"="(1.000000*(x-0.000000)+0.000000)*1.000000", "Formula From Output"="(y/1.000000-0.000000)/1.000000+0.000000"}}, {"Analog Input Channel"={"Input Type"=enum."DAQ", "Channel Name"="Window 1 to 4 dP", "Physical Channel"="cDAQ1Mod2/ai2", "Sensor Type"=enum."Differential Pressure", "Signal Type"=enum."Current", "Terminal Configuration"=-1, "Minimum Value"=0.004, "Maximum Value"=0.02, "TC Type"=10086, "Sensor Min"=0.0, "Sensor Max"=20.0, "Sensor Offset"=0.0, "Sensor Unit"=enum."inH2O", "Output Unit"=enum."Pa", "Unit Conversion"=248.84, "Active"=TRUE}, "Analog Data"={"Label"="Window1to4dP", "Offset"=0.0, "Raw"=[], "Converted"=[], "Average"=0.0, "Formula To Output"="(1250.000000*(x-0.004000)+0.000000)*248.840000", "Formula From Output"="(y/248.840000-0.000000)/1250.000000+0.004000"}}, {"Analog Input Channel"={"Input Type"=enum."DAQ", "Channel Name"="Window 1 to 7 dP", "Physical Channel"="cDAQ1Mod2/ai1", "Sensor Type"=enum."Differential Pressure", "Signal Type"=enum."Current", "Terminal Configuration"=-1, "Minimum Value"=0.004, "Maximum Value"=0.02, "TC Type"=10086, "Sensor Min"=0.0, "Sensor Max"=20.0, "Sensor Offset"=0.0, "Sensor Unit"=enum."inH2O", "Output Unit"=enum."Pa", "Unit Conversion"=248.84, "Active"=TRUE}, "Analog Data"={"Label"="Window1to7dP", "Offset"=0.0, "Raw"=[], "Converted"=[], "Average"=0.0, "Formula To Output"="(1250.000000*(x-0.004000)+0.000000)*248.840000", "Formula From Output"="(y/248.840000-0.000000)/1250.000000+0.004000"}}, {"Analog Input Channel"={"Input Type"=enum."DAQ", "Channel Name"="Window 1 to 7 Fast dP", "Physical Channel"="cDAQ1Mod2/ai0", "Sensor Type"=enum."Differential Pressure", "Signal Type"=enum."Current", "Terminal Configuration"=-1, "Minimum Value"=0.004, "Maximum Value"=0.02, "TC Type"=10086, "Sensor Min"=0.0, "Sensor Max"=2.5, "Sensor Offset"=0.0, "Sensor Unit"=enum."psi", "Output Unit"=enum."Pa", "Unit Conversion"=6894.75729, "Active"=TRUE}, "Analog Data"={"Label"="Window1to7FastdP", "Offset"=0.0, "Raw"=[], "Converted"=[], "Average"=0.0, "Formula To Output"="(156.250000*(x-0.004000)+0.000000)*6894.757290", "Formula From Output"="(y/6894.757290-0.000000)/156.250000+0.004000"}}, {"Analog Input Channel"={"Input Type"=enum."DAQ", "Channel Name"="Camera Voltage", "Physical Channel"="cDAQ1Mod8/ai0", "Sensor Type"=enum."Other", "Signal Type"=enum."Voltage", "Terminal Configuration"=10106, "Minimum Value"=0.0, "Maximum Value"=10.0, "TC Type"=10086, "Sensor Min"=0.0, "Sensor Max"=50.0, "Sensor Offset"=0.0, "Sensor Unit"=enum."Volt", "Output Unit"=enum."Volt", "Unit Conversion"=1.0, "Active"=TRUE}, "Analog Data"={"Label"="CameraVoltage", "Offset"=0.0, "Raw"=[], "Converted"=[], "Average"=0.0, "Formula To Output"="(5.000000*(x-0.000000)+0.000000)*1.000000", "Formula From Output"="(y/1.000000-0.000000)/5.000000+0.000000"}}, {"Analog Input Channel"={"Input Type"=enum."DAQ", "Channel Name"="Tinlet", "Physical Channel"="cDAQ1Mod6/ai4", "Sensor Type"=enum."Temperature", "Signal Type"=enum."Temperature", "Terminal Configuration"=-1, "Minimum Value"=0.0, "Maximum Value"=100.0, "TC Type"=10055, "Sensor Min"=-0.432, "Sensor Max"=99.438, "Sensor Offset"=0.0, "Sensor Unit"=enum."C", "Output Unit"=enum."C", "Unit Conversion"=1.0, "Active"=TRUE}, "Analog Data"={"Label"="Tinlet", "Offset"=0.0, "Raw"=[], "Converted"=[], "Average"=0.0, "Formula To Output"="(0.998700*(x-0.000000)+-0.432000)*1.000000", "Formula From Output"="(y/1.000000--0.432000)/0.998700+0.000000"}}, {"Analog Input Channel"={"Input Type"=enum."DAQ", "Channel Name"="Tsectwo", "Physical Channel"="cDAQ1Mod6/ai5", "Sensor Type"=enum."Temperature", "Signal Type"=enum."Temperature", "Terminal Configuration"=-1, "Minimum Value"=0.0, "Maximum Value"=100.0, "TC Type"=10055, "Sensor Min"=-0.3803, "Sensor Max"=99.4597, "Sensor Offset"=0.0, "Sensor Unit"=enum."C", "Output Unit"=enum."C", "Unit Conversion"=1.0, "Active"=TRUE}, "Analog Data"={"Label"="Tsectwo", "Offset"=0.0, "Raw"=[], "Converted"=[], "Average"=0.0, "Formula To Output"="(0.998400*(x-0.000000)+-0.380300)*1.000000", "Formula From Output"="(y/1.000000--0.380300)/0.998400+0.000000"}}, {"Analog Input Channel"={"Input Type"=enum."DAQ", "Channel Name"="TS Window 1 Absolute Pressure", "Physical Channel"="cDAQ1Mod5/ai12", "Sensor Type"=enum."Absolute Pressure", "Signal Type"=enum."Voltage", "Terminal Configuration"=10078, "Minimum Value"=0.0, "Maximum Value"=5.0, "TC Type"=10086, "Sensor Min"=0.0, "Sensor Max"=50.0, "Sensor Offset"=0.0, "Sensor Unit"=enum."psi", "Output Unit"=enum."Pa", "Unit Conversion"=6894.75729, "Active"=TRUE}, "Analog Data"={"Label"="TSWindow1AbsolutePressure", "Offset"=0.0, "Raw"=[], "Converted"=[], "Average"=0.0, "Formula To Output"="(10.000000*(x-0.000000)+0.000000)*6894.757290", "Formula From Output"="(y/6894.757290-0.000000)/10.000000+0.000000"}}, {"Analog Input Channel"={"Input Type"=enum."DAQ", "Channel Name"="TS Window 7 Absolute Pressure", "Physical Channel"="cDAQ1Mod5/ai13", "Sensor Type"=enum."Absolute Pressure", "Signal Type"=enum."Voltage", "Terminal Configuration"=10078, "Minimum Value"=0.0, "Maximum Value"=5.0, "TC Type"=10086, "Sensor Min"=0.0, "Sensor Max"=50.0, "Sensor Offset"=0.0, "Sensor Unit"=enum."psi", "Output Unit"=enum."Pa", "Unit Conversion"=6894.75729, "Active"=TRUE}, "Analog Data"={"Label"="TSWindow7AbsolutePressure", "Offset"=0.0, "Raw"=[], "Converted"=[], "Average"=0.0, "Formula To Output"="(10.000000*(x-0.000000)+0.000000)*6894.757290", "Formula From Output"="(y/6894.757290-0.000000)/10.000000+0.000000"}}, {"Analog Input Channel"={"Input Type"=enum."DAQ", "Channel Name"="Liquid Main Diode", "Physical Channel"="cDAQ1Mod10/ai0", "Sensor Type"=enum."Other", "Signal Type"=enum."Voltage", "Terminal Configuration"=10106, "Minimum Value"=0.0, "Maximum Value"=10.0, "TC Type"=10086, "Sensor Min"=0.0, "Sensor Max"=10.0, "Sensor Offset"=0.0, "Sensor Unit"=enum."Volt", "Output Unit"=enum."Volt", "Unit Conversion"=1.0, "Active"=TRUE}, "Analog Data"={"Label"="LiquidMainDiode", "Offset"=0.0, "Raw"=[], "Converted"=[], "Average"=0.0, "Formula To Output"="(1.000000*(x-0.000000)+0.000000)*1.000000", "Formula From Output"="(y/1.000000-0.000000)/1.000000+0.000000"}}, {"Analog Input Channel"={"Input Type"=enum."DAQ", "Channel Name"="Liquid Control Diode", "Physical Channel"="cDAQ1Mod10/ai1", "Sensor Type"=enum."Other", "Signal Type"=enum."Voltage", "Terminal Configuration"=10106, "Minimum Value"=0.0, "Maximum Value"=10.0, "TC Type"=10086, "Sensor Min"=0.0, "Sensor Max"=10.0, "Sensor Offset"=0.0, "Sensor Unit"=enum."Volt", "Output Unit"=enum."Volt", "Unit Conversion"=1.0, "Active"=TRUE}, "Analog Data"={"Label"="LiquidControlDiode", "Offset"=0.0, "Raw"=[], "Converted"=[], "Average"=0.0, "Formula To Output"="(1.000000*(x-0.000000)+0.000000)*1.000000", "Formula From Output"="(y/1.000000-0.000000)/1.000000+0.000000"}}, {"Analog Input Channel"={"Input Type"=enum."DAQ", "Channel Name"="Vapor Main Diode", "Physical Channel"="cDAQ1Mod10/ai2", "Sensor Type"=enum."Other", "Signal Type"=enum."Voltage", "Terminal Configuration"=10106, "Minimum Value"=0.0, "Maximum Value"=10.0, "TC Type"=10086, "Sensor Min"=0.0, "Sensor Max"=10.0, "Sensor Offset"=0.0, "Sensor Unit"=enum."Volt", "Output Unit"=enum."Volt", "Unit Conversion"=1.0, "Active"=TRUE}, "Analog Data"={"Label"="VaporMainDiode", "Offset"=0.0, "Raw"=[], "Converted"=[], "Average"=0.0, "Formula To Output"="(1.000000*(x-0.000000)+0.000000)*1.000000", "Formula From Output"="(y/1.000000-0.000000)/1.000000+0.000000"}}, {"Analog Input Channel"={"Input Type"=enum."DAQ", "Channel Name"="Vapor Control Diode", "Physical Channel"="cDAQ1Mod10/ai3", "Sensor Type"=enum."Other", "Signal Type"=enum."Voltage", "Terminal Configuration"=10106, "Minimum Value"=0.0, "Maximum Value"=10.0, "TC Type"=10086, "Sensor Min"=0.0, "Sensor Max"=10.0, "Sensor Offset"=0.0, "Sensor Unit"=enum."Volt", "Output Unit"=enum."Volt", "Unit Conversion"=1.0, "Active"=TRUE}, "Analog Data"={"Label"="VaporControlDiode", "Offset"=0.0, "Raw"=[], "Converted"=[], "Average"=0.0, "Formula To Output"="(1.000000*(x-0.000000)+0.000000)*1.000000", "Formula From Output"="(y/1.000000-0.000000)/1.000000+0.000000"}}, {"Analog Input Channel"={"Input Type"=enum."DAQ", "Channel Name"="TS Exterior Temperature", "Physical Channel"="cDAQ1Mod6/ai6", "Sensor Type"=enum."Temperature", "Signal Type"=enum."Temperature", "Terminal Configuration"=-1, "Minimum Value"=0.0, "Maximum Value"=100.0, "TC Type"=10073, "Sensor Min"=-0.2775, "Sensor Max"=100.1225, "Sensor Offset"=0.0, "Sensor Unit"=enum."C", "Output Unit"=enum."C", "Unit Conversion"=1.0, "Active"=TRUE}, "Analog Data"={"Label"="TSExteriorTemperature", "Offset"=0.0, "Raw"=[], "Converted"=[], "Average"=0.0, "Formula To Output"="(1.004000*(x-0.000000)+-0.277500)*1.000000", "Formula From Output"="(y/1.000000--0.277500)/1.004000+0.000000"}}, {"Analog Input Channel"={"Input Type"=enum."DAQ", "Channel Name"="DS Exterior Temperature", "Physical Channel"="cDAQ1Mod6/ai7", "Sensor Type"=enum."Temperature", "Signal Type"=enum."Temperature", "Terminal Configuration"=-1, "Minimum Value"=0.0, "Maximum Value"=100.0, "TC Type"=10073, "Sensor Min"=0.0, "Sensor Max"=100.0, "Sensor Offset"=0.0, "Sensor Unit"=enum."C", "Output Unit"=enum."C", "Unit Conversion"=1.0, "Active"=TRUE}, "Analog Data"={"Label"="DSExteriorTemperature", "Offset"=0.0, "Raw"=[], "Converted"=[], "Average"=0.0, "Formula To Output"="(1.000000*(x-0.000000)+0.000000)*1.000000", "Formula From Output"="(y/1.000000-0.000000)/1.000000+0.000000"}}, {"Analog Input Channel"={"Input Type"=enum."DAQ", "Channel Name"="Post Mixing Tee Temperature", "Physical Channel"="cDAQ1Mod7/ai2", "Sensor Type"=enum."Temperature", "Signal Type"=enum."Temperature", "Terminal Configuration"=-1, "Minimum Value"=0.0, "Maximum Value"=100.0, "TC Type"=10073, "Sensor Min"=0.0, "Sensor Max"=1000.0, "Sensor Offset"=0.0, "Sensor Unit"=enum."Volt", "Output Unit"=enum."Volt", "Unit Conversion"=1.0, "Active"=TRUE}, "Analog Data"={"Label"="PostMixingTeeTemperature", "Offset"=0.0, "Raw"=[], "Converted"=[], "Average"=0.0, "Formula To Output"="(10.000000*(x-0.000000)+0.000000)*1.000000", "Formula From Output"="(y/1.000000-0.000000)/10.000000+0.000000"}}, {"Analog Input Channel"={"Input Type"=enum."DAQ", "Channel Name"="Tsecthree", "Physical Channel"="cDAQ1Mod6/ai8", "Sensor Type"=enum."Temperature", "Signal Type"=enum."Temperature", "Terminal Configuration"=-1, "Minimum Value"=0.0, "Maximum Value"=100.0, "TC Type"=10055, "Sensor Min"=-0.2553, "Sensor Max"=99.6347, "Sensor Offset"=0.0, "Sensor Unit"=enum."C", "Output Unit"=enum."C", "Unit Conversion"=1.0, "Active"=TRUE}, "Analog Data"={"Label"="Tsecthree", "Offset"=0.0, "Raw"=[], "Converted"=[], "Average"=0.0, "Formula To Output"="(0.998900*(x-0.000000)+-0.255300)*1.000000", "Formula From Output"="(y/1.000000--0.255300)/0.998900+0.000000"}}, {"Analog Input Channel"={"Input Type"=enum."DAQ", "Channel Name"="Toutlet", "Physical Channel"="cDAQ1Mod6/ai9", "Sensor Type"=enum."Temperature", "Signal Type"=enum."Temperature", "Terminal Configuration"=-1, "Minimum Value"=0.0, "Maximum Value"=100.0, "TC Type"=10055, "Sensor Min"=-0.09939, "Sensor Max"=99.6221, "Sensor Offset"=0.0, "Sensor Unit"=enum."C", "Output Unit"=enum."C", "Unit Conversion"=1.0, "Active"=TRUE}, "Analog Data"={"Label"="Toutlet", "Offset"=0.0, "Raw"=[], "Converted"=[], "Average"=0.0, "Formula To Output"="(0.997215*(x-0.000000)+-0.099390)*1.000000", "Formula From Output"="(y/1.000000--0.099390)/0.997215+0.000000"}}] {"Analog Input Channel"."Unit Conversion" format="%0.5f"; "Analog Input Channel"."TC Type" items=["J"=10072, "K"=10073, "N"=10077, "R"=10082, "S"=10085, "T"=10086, "B"=10047, "E"=10055]; "Analog Input Channel"."Sensor Offset" format="%0.5f"; "Analog Input Channel"."Sensor Max" format="%0.5f"; "Analog Input Channel"."Sensor Min" format="%0.5f"; "Analog Input Channel"."Maximum Value" format="%.6f"; "Analog Input Channel"."Minimum Value" format="%.6f"; "Analog Input Channel"."Terminal Configuration" items=["Default"=-1, "RSE"=10083, "NRSE"=10078, "Differential"=10106, "Pseudodifferential"=12529]}, 3 "task out":refnum<k21>="input_channels")   [LabVIEW 2022 SP3]
uses:
  input_channel.ctl
  analog_data_channel_pkg.ctl
  analog_data.ctl
  <vilib>/DAQmx/create/channels.llb/DAQmx Create Channel (AI-Current-Basic).vi
  <vilib>/DAQmx/create/channels.llb/DAQmx Create Channel (AI-Voltage-Basic).vi
  <vilib>/DAQmx/create/channels.llb/DAQmx Create Channel (AI-Temperature-Thermocouple).vi
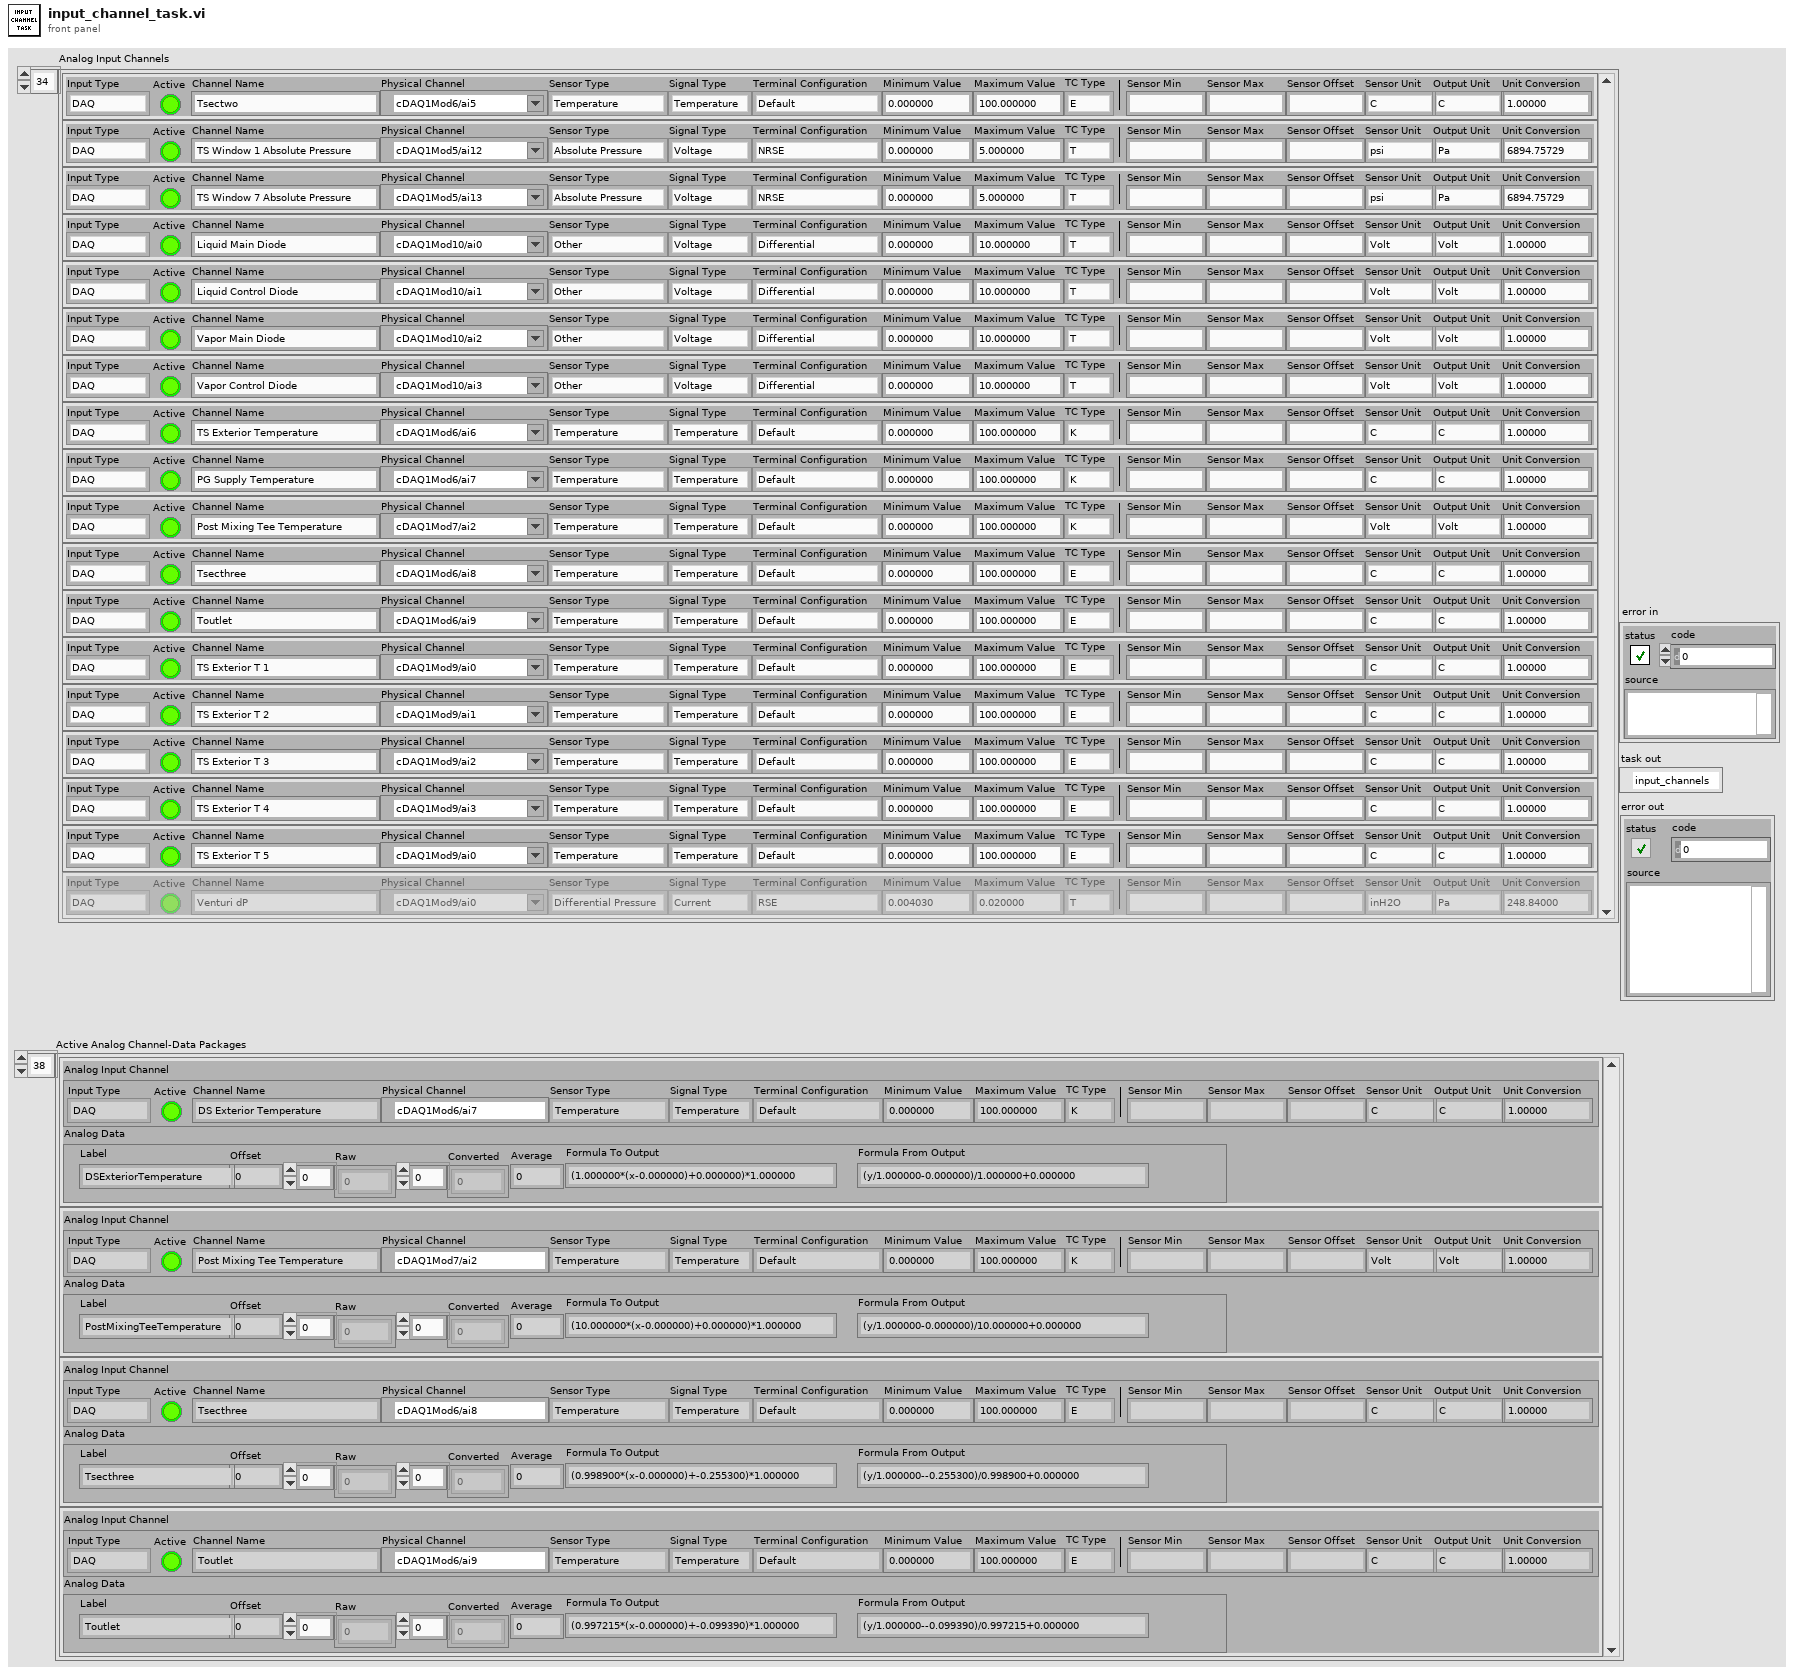
[diagram p1: front panel]
types:
  T1 = typedef "analog_data_channel_pkg.ctl" = cluster{"Analog Input Channel":T2, "Analog Data":T3}
  T2 = typedef "input_channel.ctl" = cluster{"Input Type":enum16{"DAQ", "Add-On"}, "Channel Name":string, "Physical Channel":tag, "Sensor Type":enum16{"Absolute Pressure", "Gauge Pressure", "Differential Pressure", "Temperature", "Mass Flow Rate", "Density", "Other"}, "Signal Type":enum16{"Voltage", "Current", "Temperature"}, "Terminal Configuration":i32, "Minimum Value":dbl, "Maximum Value":dbl, "TC Type":i32, "Sensor Min":dbl, "Sensor Max":dbl, "Sensor Offset":dbl, "Sensor Unit":enum16{"psi", "Pa", "inH2O", "inHg", "C", "K", "g/s", "g/cm3", "Volt", "Amp", ""}, "Output Unit":enum16{"psi", "Pa", "inH2O", "inHg", "C", "K", "g/s", "g/cm3", "Volt", "Amp", ""}, "Unit Conversion":dbl, "Active":bool}
  T3 = typedef "analog_data.ctl" = cluster{"Label":string, "Offset":dbl, "Raw":dbl[], "Converted":dbl[], "Average":dbl, "Formula To Output":string, "Formula From Output":string}
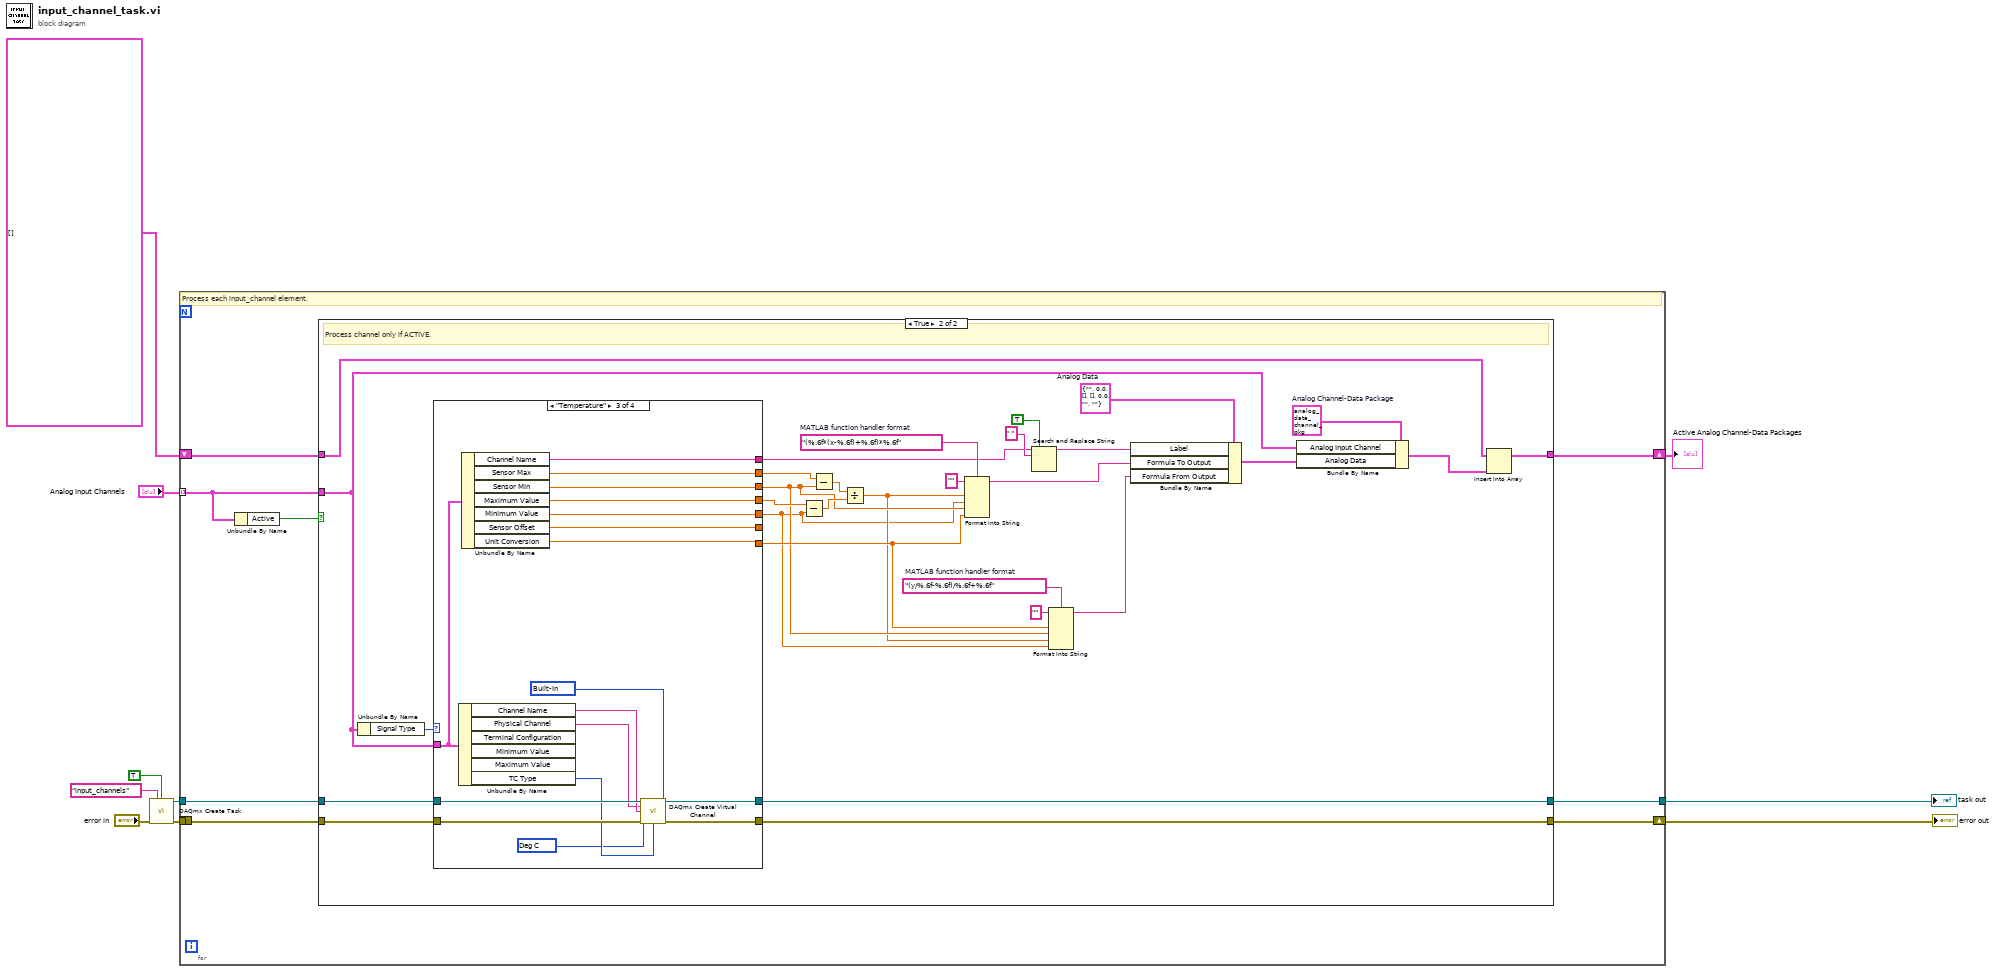
[diagram p0: block diagram]
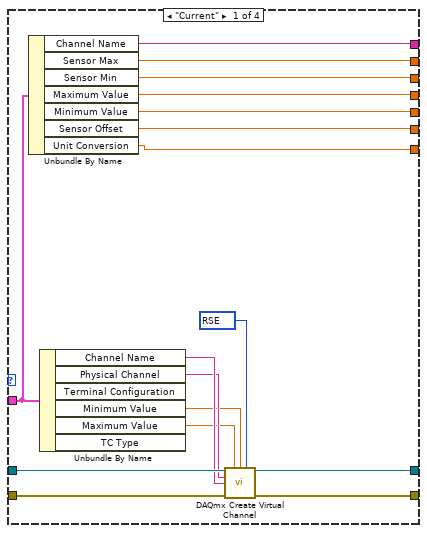
[diagram p3: hidden frame]
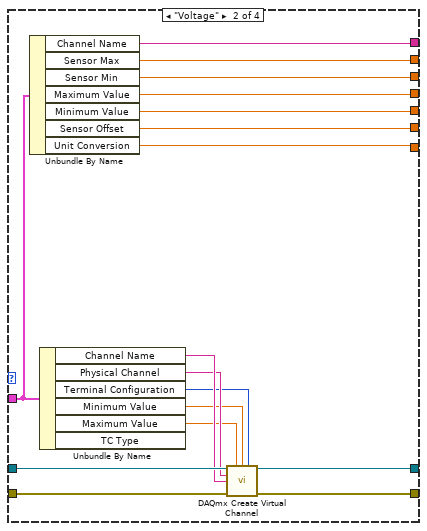
[diagram p4: hidden frame]
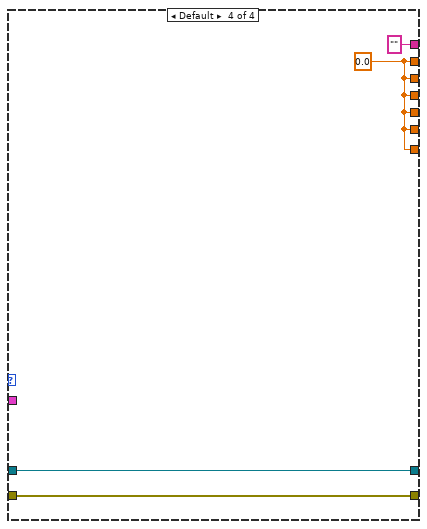
[diagram p5: hidden frame]
diagram:
  n1 = call <vilib>:"DAQmx Create Task.vi"("new task name"="input_channels", "auto cleanup"=TRUE, "error in"="error in") -> ("task out"=w7:refnum<k21>, "error out"=w6:errorcluster)  [unwired: 11 in]
  n2 = for {
    tunnel: "Analog Input Channels" -> [w14] mode=indexing
    tunnel: w7 -> [w18]
    tunnel: w6 -> [w17]
    tunnel: [w16] -> w4
    shift-right: [w15] -> w1
    shift-left: T1[] [] ("Array") -> [w12]
    shift-right: [w11] -> w3
    shift-left: _ -> [_]
    # "Process each input_channel element."
    n3 = Unbundle By Name(w14) -> ("Active"=w13:bool)
    n4 = case shown="True" w13 {
      tunnel: w18 -> [w21 w50]
      tunnel: w17 -> [w20 w49]
      tunnel: [w21 w48] -> w16
      tunnel: [w20 w23] -> w11
      tunnel: w14 -> [_ w28]
      tunnel: [w19 w25] -> w15
      tunnel: w12 -> [w19 w26]
      frame False {
        # "Skip Channel if NOT ACTIVE."
      }
      frame True {
        w30 = T1 {"Analog Input Channel"={"Input Type"=enum."DAQ", "Channel Name"="", "Physical Channel"="", "Sensor Type"=enum."Absolute Pressure", "Signal Type"=enum."Voltage", "Terminal Configuration"=-1, "Minimum Value"=5.0, "Maximum Value"=5.0, "TC Type"=10072, "Sensor Min"=5.0, "Sensor Max"=5.0, "Sensor Offset"=5.0, "Sensor Unit"=enum."psi", "Output Unit"=enum."psi", "Unit Conversion"=5.0, "Active"=TRUE}, "Analog Data"={"Label"="", "Offset"=0.0, "Raw"=[], "Converted"=[], "Average"=0.0, "Formula To Output"="", "Formula From Output"=""}}  # Analog Channel-Data Package
        w37 = "(y/%.6f-%.6f)/%.6f+%.6f"  # MATLAB function handler format
        w47 = T3 {"Label"="", "Offset"=0.0, "Raw"=[], "Converted"=[], "Average"=0.0, "Formula To Output"="", "Formula From Output"=""}  # Analog Data
        w40 = "(%.6f*(x-%.6f)+%.6f)*%.6f"  # MATLAB function handler format
        # "Process channel only if ACTIVE."
        n5 = Unbundle By Name(w28) -> ("Signal Type"=w51:enum16{"Voltage", "Current", "Temperature"})
        n6 = case shown="\"Temperature\"" w51 {
          tunnel: w50 -> [w68 w85 w100 w106]
          tunnel: w49 -> [w67 w82 w99 w105]
          tunnel: [w64 w84 w102 w106] -> w48
          tunnel: [w63 w83 w101 w105] -> w23
          tunnel: w28 -> [w56 w71 w95 _]
          tunnel: [w62 w77 w94 "" ("Channel Name")] -> w27
          tunnel: [w61 w76 w93 w103] -> w22
          tunnel: [w60 w75 w92 w103] -> w33
          tunnel: [w59 w74 w91 w103] -> w43
          tunnel: [w58 w73 w90 w103] -> w31
          tunnel: [w57 w72 w89 w103] -> _
          tunnel: [w55 w70 w88 w103] -> w34
          frame "Current" {
            w52 = 10083 items=["default"=-1, "RSE"=10083, "NRSE"=10078, "Differential"=10106, "Pseudodifferential"=12529] ("input terminal configuration")
            n7 = Unbundle By Name(w56) -> ("Channel Name"=w62:string, "Sensor Max"=w61:dbl, "Sensor Min"=w60:dbl, "Maximum Value"=w59:dbl, "Minimum Value"=w58:dbl, "Sensor Offset"=w57:dbl, "Unit Conversion"=w55:dbl)
            n8 = Unbundle By Name(w56) -> ("Channel Name"=w66:string, "Physical Channel"=w65:tag, "Minimum Value"=w54:dbl, "Maximum Value"=w53:dbl)  [unwired: 2 out]
            n9 = call-poly <vilib>:"DAQmx Create Virtual Channel.vi"("task in"=w68, "maximum value"=w53, "minimum value"=w54, "input terminal configuration"=w52, "physical channels"=w65, "name to assign"=w66, "error in"=w67) -> ("task out"=w64:refnum<k21>, "error out"=w63:errorcluster)  [unwired: 7 in]
          }
          frame "Voltage" {
            n10 = Unbundle By Name(w71) -> ("Channel Name"=w77:string, "Sensor Max"=w76:dbl, "Sensor Min"=w75:dbl, "Maximum Value"=w74:dbl, "Minimum Value"=w73:dbl, "Sensor Offset"=w72:dbl, "Unit Conversion"=w70:dbl)
            n11 = Unbundle By Name(w71) -> ("Channel Name"=w81:string, "Physical Channel"=w80:tag, "Terminal Configuration"=w69:i32, "Minimum Value"=w79:dbl, "Maximum Value"=w78:dbl)  [unwired: 1 out]
            n12 = call-poly <vilib>:"DAQmx Create Virtual Channel.vi"("task in"=w85, "maximum value"=w78, "minimum value"=w79, "input terminal configuration"=w69, "physical channels"=w80, "name to assign"=w81, "error in"=w82) -> ("task out"=w84:refnum<k21>, "error out"=w83:errorcluster)  [unwired: 7 in]
          }
          frame "Temperature" {
            w86 = 10200 items=["Built-In"=10200, "Constant Value"=10116, "Channel"=10113] ("cjc source")
            w87 = 10143 items=["Deg C"=10143, "Deg F"=10144, "Kelvins"=10325, "Deg R"=10145, "From Custom Scale"=10065] ("units")
            n13 = Unbundle By Name(w95) -> ("Channel Name"=w97:string, "Physical Channel"=w96:tag, "TC Type"=w98:i32)  [unwired: 3 out]
            n14 = Unbundle By Name(w95) -> ("Channel Name"=w94:string, "Sensor Max"=w93:dbl, "Sensor Min"=w92:dbl, "Maximum Value"=w91:dbl, "Minimum Value"=w90:dbl, "Sensor Offset"=w89:dbl, "Unit Conversion"=w88:dbl)
            n15 = call-poly <vilib>:"DAQmx Create Virtual Channel.vi"("task in"=w100, "physical channels"=w96, "cjc source"=w86, "name to assign"=w97, "units"=w87, "error in"=w99, "thermocouple type"=w98) -> ("task out"=w102:refnum<k21>, "error out"=w101:errorcluster)  [unwired: 7 in]
          }
          frame Default {
            w103 = 0.0
          }
        }
        n16 = Subtract(x=w43, y=w31) -> (x-y=w42:dbl)
        n17 = Subtract(x=w22, y=w33) -> (x-y=w41:dbl)
        n18 = Divide(x=w41, y=w42) -> (x/y=w32:dbl)
        n19 = Format Into String(format string=w40, initial string="", w32, w31, w33, w34) -> (resulting string=w38:string)  [unwired: 1 in, 1 out]
        n20 = Search and Replace String(replace all?=TRUE ("replace all? (F)"), input string=w27, search string=" ") -> (result string=w44:string)  [unwired: 5 in, 3 out]
        n21 = Format Into String(format string=w37, initial string="", w34, w33, w32, w31) -> (resulting string=w35:string)  [unwired: 1 in, 1 out]
        n22 = Bundle By Name(cluster=w47, "Label"=w44, "Formula To Output"=w38, "Formula From Output"=w35) -> (w29:T3)
        n23 = Bundle By Name(cluster=w30, "Analog Input Channel"=w28, "Analog Data"=w29) -> (w24:T1)
        n24 = Insert Into Array(array=w26, new element=w24) -> (w25:T1[])  [unwired: 1 in]
      }
    }
  }
  "task out" <- w4
  "error out" <- w3
  "Active Analog Channel-Data Packages" <- w1
